vi "Build Port Array.vi"(8 "error in (no error)":errorcluster, 11 "DAQmxDI in":refnum<class "DAQmxDI.lvclass">) -> (0 "error out":errorcluster, 3 "DAQmxDI out":refnum<class "DAQmxDI.lvclass">)   [LabVIEW 2020, in "VolatusDAQ.lvlib" / "DAQmxDI.lvclass"]
uses:
  DAQmxDI.lvclass
  DAQmxDI.lvclass/DAQmxDI.ctl
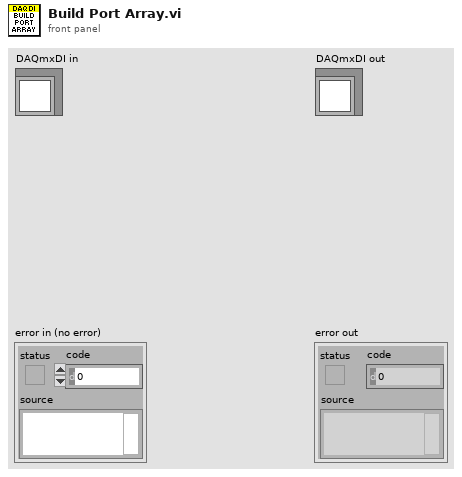
[diagram p1: front panel]
types:
  T1 = typedef "VolatusDAQ.lvlib/DAQmxDI.lvclass/Port Info.ctl" = cluster{"Module Alias":string, "Number":i32, "# Lines":i32, "Lines":map{i32, string}, "Channel Indices":i32[]}
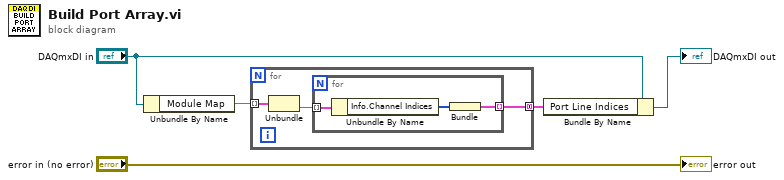
[diagram p0: block diagram]
diagram:
  n1 = Unbundle By Name("DAQmxDI in") -> ("Module Map"=w3:map{string, map{i32, T1}})
  n2 = for {
    tunnel: w3 -> [w8] mode=indexing
    tunnel: [w6] -> w1 mode=concatenating
    n3 = Unbundle(w8) -> ("Ports"=w7:map{i32, T1})  [unwired: 1 out]
    n4 = for {
      tunnel: w7 -> [w11] mode=indexing
      tunnel: [w9] -> w6 mode=indexing
      n5 = Unbundle By Name(w11) -> ("Info.Channel Indices"=w10:i32[])
      n6 = Bundle("Channel Indices"=w10) -> (w9:cluster{"Channel Indices":i32[]})  [unwired: 1 in]
    }
  }
  n7 = Bundle By Name(cluster="DAQmxDI in", "Port Line Indices"=w1) -> (→"DAQmxDI out":refnum<class "DAQmxDI.lvclass">)
  "error out" <- "error in (no error)"
